vi "xy振镜移动-v2.vi"(0 "AO通道：X前Y后":tag="Dev1/ao0:1", 1 "f_scanlens(mm)":dbl=50.0, 2 "f_tubelens(mm)":dbl=200.0, 3 "f_objecitve(mm)":dbl=1.8, 5 "x终止位(um)":dbl=10.0, 7 "y终止位(um)":dbl=10.0, 9 "x初始位(um)":dbl, 11 "y初始位(um)":dbl, 12 "速度(um/s)":dbl=10.0, 13 "比例因子(V/°)":dbl=0.5) -> (6 "x终止位(um) 2":dbl=10.0, 8 "y终止位(um) 2":dbl=10.0)   [LabVIEW 2015]
doc: "速度为0时执行G0指令，可无需连接XY初始角"
uses:
  <vilib>/Platform/TimedLoop/XDataNode/timing_clust.ctl
  <vilib>/Platform/TimedLoop/XDataNode/nitl_modes.ctl
  <vilib>/Platform/TimedLoop/XDataNode/wakeup.ctl
  <vilib>/DAQmx/write.llb/DAQmx Write (Analog 1D DBL NChan 1Samp).vi
  <vilib>/DAQmx/write.llb/DAQmx Write (Analog DBL 1Chan 1Samp).vi
  <vilib>/DAQmx/create/channels.llb/DAQmx Create Channel (AO-Voltage-Basic).vi
  <vilib>/DAQmx/miscellaneous.llb/DAQmx Fill In Error Info.vi
  <vilib>/Platform/TimedLoop/XDataNode/XDataNode.xnode
  <vilib>/Platform/TimedLoop/XDataNode/XDNodeRunTimeDep.lvlib
panel:
  out "x当前角度(°)":dbl
  out "xy当前角度(°)":dbl[](array[numeric])
  out "y变压轨迹(°)":dbl[](array[numeric])=[0.0, 0.0, 0.002017457026776073, 0.006052371120349187, 0.012104742510839941, 0.020174571918626052, 0.030261861004579515, 0.042366612970385624, 0.05648883330894886, 0.07262853070489507, 0.09078571808518568, 0.11096041381986907, 0.13315264307300606, 0.15736243930382154, 0.1835898459181542, 0.21183491807029903, 0.24209772461536572, 0.27437835021230905, 0.30867689757782557, 0.3449934898913579, 0.38332827335149355, 0.42368141988411046, 0.46605313000267945, 0.5104436358212108, 0.5568532042204127, 0.6052821401677164, 0.6557307901919239, 0.7081995460133446, 0.7626888483303975, 0.819199190763796, 0.8777311239595615, 0.9382852598522744, 1.0008622760901253, 1.0654629206235144, 1.1320880164591356, 1.2007384665816805, 1.271415259045531, 1.3441194722390282, 1.4188522803241743, 1.495614958854875, 1.5744088905771372, 1.6552355714149243, 1.7380966166457146, 1.8229937672701457, 1.909928896580496, 1.998904016933165, 2.0899212867307106, 2.18298301761946, 2.2780916819091943, 2.375249920221874, 2.4744605493769543, 2.575726570521373, 2.6790511775129087, 2.784437765566249, 2.891889940171799, 3.0014115262979684, 3.1130065778884597, 3.226679387666904, 3.3424344972620594, 3.4602767076677168, 3.5802110900524586, 3.702242996935469, 3.826378073745729, 3.952622270783123, 4.080981855601287, 4.211463425833395, 4.344073922483553, 4.478820643708048, 4.615711259112385, 4.754753824591847, 4.895956797745277, 5.039329053893832, 5.18487990273871, 5.3326191056942776, 5.4825568939355716, 5.6347039872019975, 5.789071613401982, 5.94567152906667, 6.1045160407041665, 6.265618027109712, 6.428990962691198, 6.5946489418739285, 6.762606704653315, 6.932879663369455, 7.105483930783171, 7.2804363495393325, 7.4577545231099505, 7.6374568483168614, 7.819562549541885, 8.004091714740943, 8.19106533338831, 8.380505336487511, 8.572434638796867, 8.766877183430273, 8.963857989007577, 9.163403199544092, 9.365540137285489, 9.570297358712834, 9.777704713962741, 9.987793409930267, 10.200596077346972, 10.416146842154335, 10.634481401523217, 10.855637104904389, 11.079653040532992, 11.306570127852297, 11.536431216369454, 11.769281191509043, 12.00516708808958, 12.244138212115095, 12.486246271648975, 12.731545517622042, 12.980092895522644, 13.231948209024937, 13.487174296734457, 13.745837223369977, 14.008006486859884, 14.27375524301323, 14.543160549633939, 14.816303632185644, 15.09327017338965, 15.374150629455835, 15.659040576013455, 15.948041087234744, 16.241259152139953, 16.53880813265128, 16.84080826864106, 17.14738723601639, 17.45868076482219, 17.774833325457493, 18.095998892422205, 18.42234179659009, 18.754037678895433, 19.09127456059879, 19.434254048052267, 19.783192693234888, 20.13832353542236, 20.499897854386717, 20.868187171740544, 21.24348554477633, 21.62611220683683, 22.01641462046435, 22.4147720250887]
  out "x变压轨迹(°)":dbl[](array[numeric])=[0.0, 0.0, 0.002017457026776073, 0.006052371120349187, 0.012104742510839941, 0.020174571918626052, 0.030261861004579515, 0.042366612970385624, 0.05648883330894886, 0.07262853070489507, 0.09078571808518568, 0.11096041381986907, 0.13315264307300606, 0.15736243930382154, 0.1835898459181542, 0.21183491807029903, 0.24209772461536572, 0.27437835021230905, 0.30867689757782557, 0.3449934898913579, 0.38332827335149355, 0.42368141988411046, 0.46605313000267945, 0.5104436358212108, 0.5568532042204127, 0.6052821401677164, 0.6557307901919239, 0.7081995460133446, 0.7626888483303975, 0.819199190763796, 0.8777311239595615, 0.9382852598522744, 1.0008622760901253, 1.0654629206235144, 1.1320880164591356, 1.2007384665816805, 1.271415259045531, 1.3441194722390282, 1.4188522803241743, 1.495614958854875, 1.5744088905771372, 1.6552355714149243, 1.7380966166457146, 1.8229937672701457, 1.909928896580496, 1.998904016933165, 2.0899212867307106, 2.18298301761946, 2.2780916819091943, 2.375249920221874, 2.4744605493769543, 2.575726570521373, 2.6790511775129087, 2.784437765566249, 2.891889940171799, 3.0014115262979684, 3.1130065778884597, 3.226679387666904, 3.3424344972620594, 3.4602767076677168, 3.5802110900524586, 3.702242996935469, 3.826378073745729, 3.952622270783123, 4.080981855601287, 4.211463425833395, 4.344073922483553, 4.478820643708048, 4.615711259112385, 4.754753824591847, 4.895956797745277, 5.039329053893832, 5.18487990273871, 5.3326191056942776, 5.4825568939355716, 5.6347039872019975, 5.789071613401982, 5.94567152906667, 6.1045160407041665, 6.265618027109712, 6.428990962691198, 6.5946489418739285, 6.762606704653315, 6.932879663369455, 7.105483930783171, 7.2804363495393325, 7.4577545231099505, 7.6374568483168614, 7.819562549541885, 8.004091714740943, 8.19106533338831, 8.380505336487511, 8.572434638796867, 8.766877183430273, 8.963857989007577, 9.163403199544092, 9.365540137285489, 9.570297358712834, 9.777704713962741, 9.987793409930267, 10.200596077346972, 10.416146842154335, 10.634481401523217, 10.855637104904389, 11.079653040532992, 11.306570127852297, 11.536431216369454, 11.769281191509043, 12.00516708808958, 12.244138212115095, 12.486246271648975, 12.731545517622042, 12.980092895522644, 13.231948209024937, 13.487174296734457, 13.745837223369977, 14.008006486859884, 14.27375524301323, 14.543160549633939, 14.816303632185644, 15.09327017338965, 15.374150629455835, 15.659040576013455, 15.948041087234744, 16.241259152139953, 16.53880813265128, 16.84080826864106, 17.14738723601639, 17.45868076482219, 17.774833325457493, 18.095998892422205, 18.42234179659009, 18.754037678895433, 19.09127456059879, 19.434254048052267, 19.783192693234888, 20.13832353542236, 20.499897854386717, 20.868187171740544, 21.24348554477633, 21.62611220683683, 22.01641462046435, 22.4147720250887]
  out "移动次数":i32=142
  in  "AO通道：单通道":tag="Dev1/ao0:1"
  in  "dt(ms)":i32=10
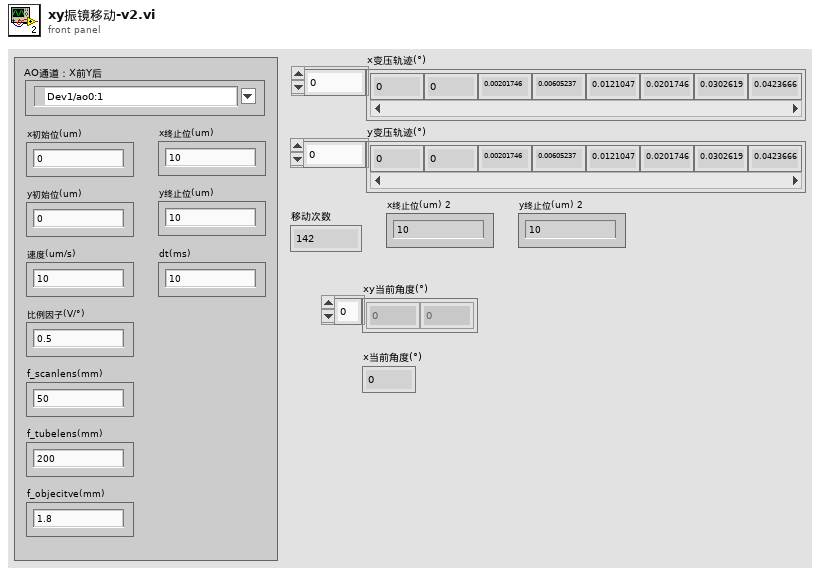
[diagram p1: front panel]
types:
  T1 = typedef "XDNodeRunTimeDep.lvlib/timing_clust.ctl" = cluster{"Expected End [f-1]":u64, "Actual End [f-1]":u64, "Finished Late? [f-1]":bool, "Expected End [i-1]":u64, "Actual End [i-1]":u64, "Finished Late? [i-1]":bool, "Expected Start [i]":u64, "Actual Start [i]":u64, "Expected Start [f]":u64, "Actual Start [f]":u64, "Source Name":string, "Structure Name":string, "Period":i64, "Deadline":i64, "Offset":i64, "Start":i64, "Priority":i32, "Timeout":i32, "Mode":T2, "Wakeup Reason":T3, "Error":errorcluster, "Source Type":string, "Secondary Source Type":string, "Global End Time":u64, "Global Start Time":u64, "Frame Duration":u64, "Iteration Duration":u64, "Assigned CPU":i32, "I/O Scan Engine Mode":u32}
  T2 = typedef "XDNodeRunTimeDep.lvlib/nitl_modes.ctl" = enum32{"No Change", "Process missed periods, maintain original phase", "Discard missed periods, maintain original phase", "Process missed periods, ignore original phase", "Discard missed periods, ignore original phase"}
  T3 = typedef "XDNodeRunTimeDep.lvlib/wakeup.ctl" = enum32{"Normal", "Aborted", "Asynchronous wakeup", "Timing source error", "Timed loop error", "Timeout"}
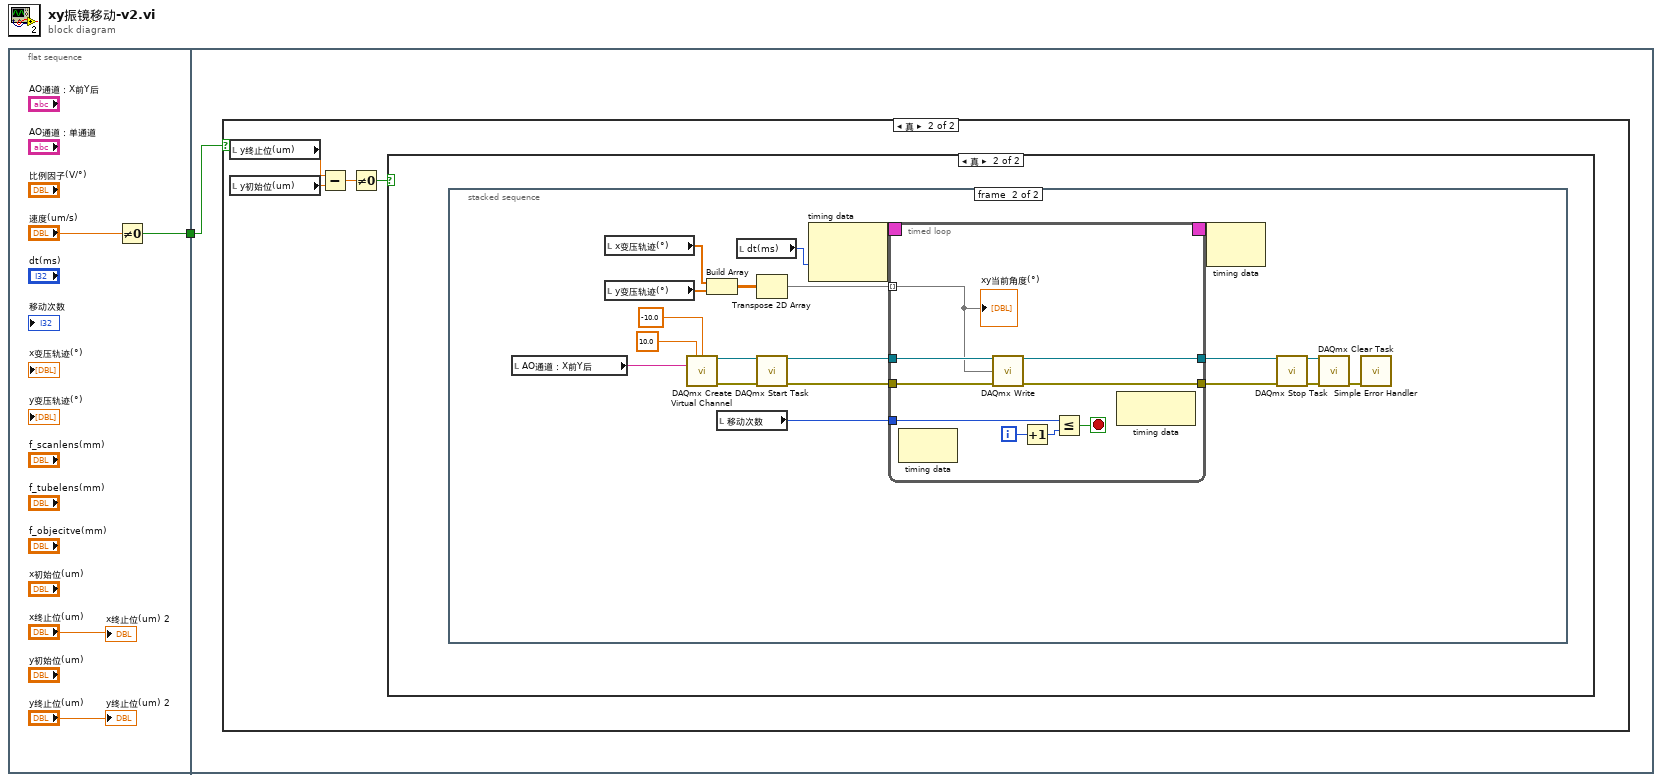
[diagram p0: block diagram]
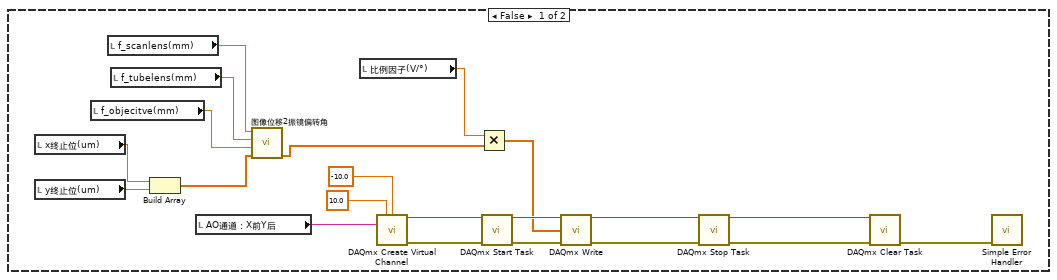
[diagram p2: hidden frame]
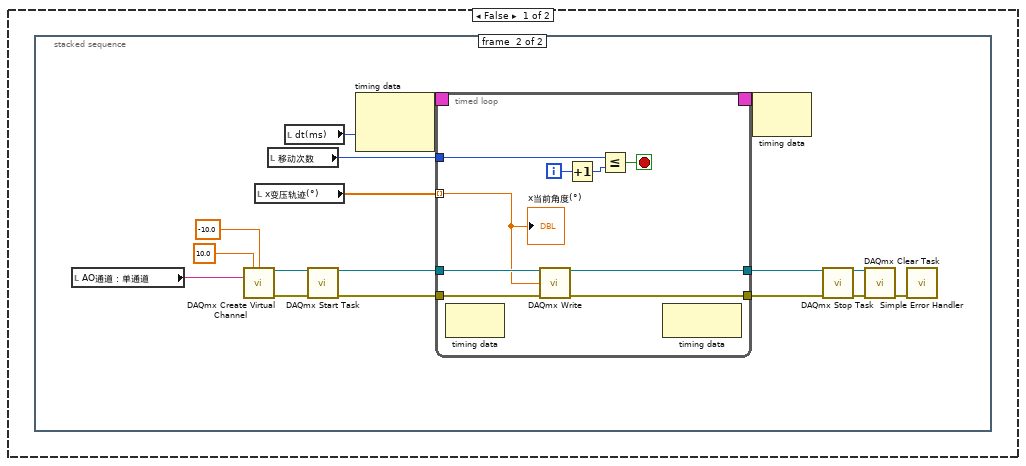
[diagram p3: hidden frame]
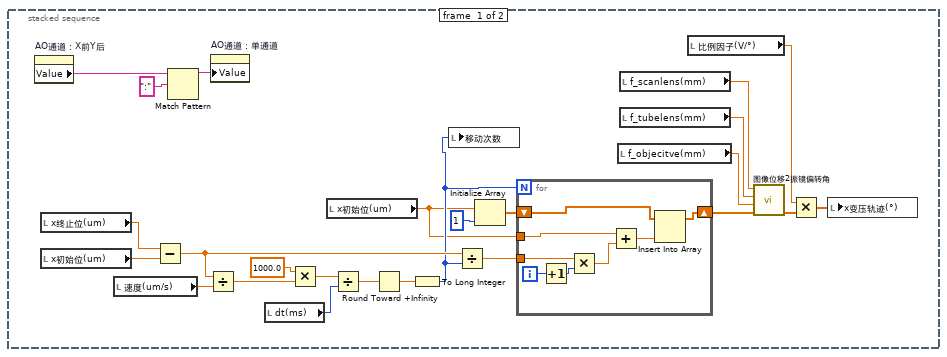
[diagram p4: hidden frame]
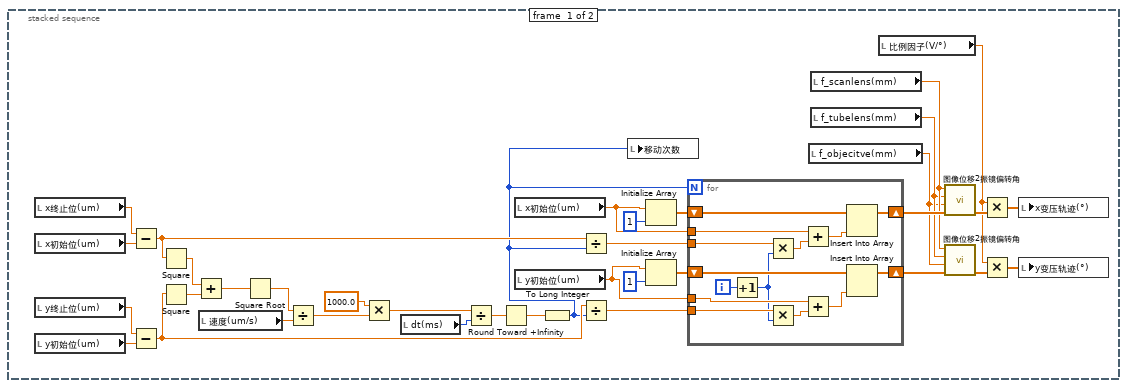
[diagram p5: hidden frame]
diagram:
  n1 = flat-sequence {
    tunnel: [w5] -> w1
    tunnel: w1 -> [w6]
    frame #0 {
      n2 = Not Equal To 0?(x="速度(um/s)") -> (x != 0?=w5:bool)
      "x终止位(um) 2" <- "x终止位(um)"
      "y终止位(um) 2" <- "y终止位(um)"
    }
    frame #1 {
      n3 = case shown="真" w6 {
        frame False {
          n4 = local read "x终止位(um)"() -> (w14:dbl)
          n5 = local read "y终止位(um)"() -> (w15:dbl)
          n6 = local read "f_objecitve(mm)"() -> (w9:dbl)
          n7 = local read "f_scanlens(mm)"() -> (w11:dbl)
          n8 = local read "f_tubelens(mm)"() -> (w10:dbl)
          n9 = Build Array(w14, w15) -> (w8:dbl[])
          n10 = local read "AO通道：X前Y后"() -> (w12:tag)
          n11 = call "图像位移2振镜偏转角.vi"("图像位移(um)"=w8, "f_objecitve(mm)"=w9, "f_tubelens(mm)"=w10, "f_scanlens(mm)"=w11) -> ("振镜偏转角(°)"=w7:dbl[])  [unwired: 7 in]
          n12 = local read "比例因子(V/°)"() -> (w13:dbl)
          n13 = call-poly <vilib>:"DAQmx Create Virtual Channel.vi"("maximum value"=10.0, "minimum value"=-10.0, "physical channels"=w12) -> ("task out"=w26:refnum<k21>, "error out"=w25:errorcluster)  [unwired: 11 in]
          n14 = Multiply(x=w13, y=w7) -> (x*y=w19:dbl[])
          n15 = call <vilib>:"DAQmx Start Task.vi"("task/channels in"=w26, "error in"=w25) -> ("task out"=w20:refnum<k21>, "error out"=w16:errorcluster)  [unwired: 12 in]
          n16 = call-poly <vilib>:"DAQmx Write.vi"("task/channels in"=w20, "data"=w19, "error in"=w16) -> ("task out"=w18:refnum<k21>, "error out"=w17:errorcluster)  [unwired: 10 in, 1 out]
          n17 = call <vilib>:"DAQmx Stop Task.vi"("task/channels in"=w18, "error in"=w17) -> ("task out"=w24:refnum<k21>, "error out"=w23:errorcluster)  [unwired: 12 in]
          n18 = call <vilib>:"DAQmx Clear Task.vi"("task in"=w24, "error in"=w23) -> ("error out"=w27:errorcluster)  [unwired: 13 in]
          n19 = call <vilib>:"Simple Error Handler.vi"("error in (no error)"=w27) -> ()  [unwired: 4 in, 5 out]
        }
        frame True {
          n20 = local read "y终止位(um)"() -> (w29:dbl)
          n21 = local read "y初始位(um)"() -> (w28:dbl)
          n22 = Subtract(x=w29, y=w28) -> (x-y=w31:dbl)
          n23 = Not Equal To 0?(x=w31) -> (x != 0?=w30:bool)
          n24 = case shown="真" w30 {
            frame False {
              n25 = stacked-sequence {
                frame #0 {
                  n26 = property on="AO通道：X前Y后" class="DAQmxName"() -> ("Value"=w54:string)  [unwired: 2 in, 2 out]
                  n27 = local read "x终止位(um)"() -> (w39:dbl)
                  n28 = local read "x初始位(um)"() -> (w41:dbl)
                  n29 = local read "速度(um/s)"() -> (w40:dbl)
                  n30 = Subtract(x=w39, y=w41) -> (x-y=w53:dbl)
                  n31 = Match Pattern(string=w54, regular expression=":" ("正则表达式")) -> (before substring=w56:string)  [unwired: 1 in, 3 out]
                  n32 = Divide(x=w53, y=w40) -> (x/y=w36:dbl)
                  n33 = property on="AO通道：单通道" class="DAQmxName"("Value"=w56) -> ()  [unwired: 2 in, 2 out]
                  n34 = local read "dt(ms)"() -> (w42:i32)
                  n35 = Multiply(x=1000.0, y=w36) -> (x*y=w38:dbl)
                  n36 = local read "x初始位(um)"() -> (w32:dbl)
                  n37 = Divide(x=w38, y=w42) -> (x/y=w34:dbl)
                  n38 = Round Toward +Infinity(x=w34) -> (ceil(x): smallest int >= x=w35:dbl)
                  n39 = To Long Integer(number=w35) -> (32bit integer=w33:i32)
                  n40 = local write "移动次数"(w33) -> ()
                  n41 = Divide(x=w53, y=w33) -> (x/y=w44:dbl)
                  n42 = Initialize Array(w32, 1 ("维数大小")) -> (w43:dbl[])
                  n43 = for {
                    N: w33 -> [_]
                    shift-right: [w60] -> w46
                    shift-left: w43 -> [w64]
                    tunnel: w44 -> [w63]
                    tunnel: w32 -> [w57]
                    i -> [w59]
                    n44 = Increment(x=w59) -> (x+1=w58:i32)
                    n45 = Multiply(x=w63, y=w58) -> (x*y=w62:dbl)
                    n46 = Add(x=w57, y=w62) -> (x+y=w61:dbl)
                    n47 = Insert Into Array(array=w64, new element=w61) -> (w60:dbl[])  [unwired: 1 in]
                  }
                  n48 = local read "f_objecitve(mm)"() -> (w49:dbl)
                  n49 = local read "f_scanlens(mm)"() -> (w47:dbl)
                  n50 = local read "f_tubelens(mm)"() -> (w48:dbl)
                  n51 = local read "比例因子(V/°)"() -> (w52:dbl)
                  n52 = call "图像位移2振镜偏转角.vi"("图像位移(um)"=w46, "f_objecitve(mm)"=w49, "f_tubelens(mm)"=w48, "f_scanlens(mm)"=w47) -> ("振镜偏转角(°)"=w50:dbl[])  [unwired: 7 in]
                  n53 = Multiply(x=w52, y=w50) -> (x*y=w51:dbl[])
                  n54 = local write "x变压轨迹(°)"(w51) -> ()
                }
                frame #1 {
                  n55 = local read "AO通道：单通道"() -> (w67:tag)
                  n56 = call-poly <vilib>:"DAQmx Create Virtual Channel.vi"("maximum value"=10.0, "minimum value"=-10.0, "physical channels"=w67) -> ("task out"=w78:refnum<k21>, "error out"=w77:errorcluster)  [unwired: 11 in]
                  n57 = local read "x变压轨迹(°)"() -> (w65:dbl[])
                  n58 = local read "移动次数"() -> (w66:i32)
                  n59 = local read "dt(ms)"() -> (w70:i32)
                  n60 = call <vilib>:"DAQmx Start Task.vi"("task/channels in"=w78, "error in"=w77) -> ("task out"=w76:refnum<k21>, "error out"=w75:errorcluster)  [unwired: 12 in]
                  n61 = node-c288(w70) -> (w81:T1)  [unwired: 1 in]
                  n62 = timed-loop {
                    tunnel: w76 -> [w90]
                    tunnel: w75 -> [w88]
                    tunnel: [w87] -> w73
                    tunnel: [w89] -> w74
                    timing: w81 -> [_]
                    timing-out: [_] -> w80
                    tunnel: w66 -> [w84]
                    tunnel: w65 -> [w82] mode=indexing
                    i -> [w86]
                    stop <- w83 stop-if-true
                    n63 = node-c288() -> ()  [unwired: 1 in, 1 out]
                    n64 = call-poly <vilib>:"DAQmx Write.vi"("task/channels in"=w90, "data"=w82, "error in"=w88) -> ("task out"=w89:refnum<k21>, "error out"=w87:errorcluster)  [unwired: 10 in, 1 out]
                    n65 = Increment(x=w86) -> (x+1=w85:i32)
                    n66 = Less Or Equal?(x=w84, y=w85) -> (x <= y?=w83:bool)
                    n67 = node-c288() -> ()  [unwired: 1 in, 1 out]
                    "x当前角度(°)" <- w82
                  }
                  n68 = node-c288(w80) -> ()  [unwired: 1 out]
                  n69 = call <vilib>:"DAQmx Stop Task.vi"("task/channels in"=w74, "error in"=w73) -> ("task out"=w72:refnum<k21>, "error out"=w71:errorcluster)  [unwired: 12 in]
                  n70 = call <vilib>:"DAQmx Clear Task.vi"("task in"=w72, "error in"=w71) -> ("error out"=w79:errorcluster)  [unwired: 13 in]
                  n71 = call <vilib>:"Simple Error Handler.vi"("error in (no error)"=w79) -> ()  [unwired: 4 in, 5 out]
                }
              }
            }
            frame True {
              n72 = stacked-sequence {
                frame #0 {
                  n73 = local read "x终止位(um)"() -> (w120:dbl)
                  n74 = local read "x初始位(um)"() -> (w117:dbl)
                  n75 = local read "y终止位(um)"() -> (w119:dbl)
                  n76 = local read "y初始位(um)"() -> (w121:dbl)
                  n77 = Subtract(x=w120, y=w117) -> (x-y=w122:dbl)
                  n78 = Subtract(x=w119, y=w121) -> (x-y=w123:dbl)
                  n79 = Square(x=w122) -> (x^2=w129:dbl)
                  n80 = Square(x=w123) -> (x^2=w130:dbl)
                  n81 = Add(x=w129, y=w130) -> (x+y=w131:dbl)
                  n82 = local read "速度(um/s)"() -> (w118:dbl)
                  n83 = Square Root(x=w131) -> (sqrt(x)=w132:dbl)
                  n84 = Divide(x=w132, y=w118) -> (x/y=w126:dbl)
                  n85 = Multiply(x=1000.0, y=w126) -> (x*y=w124:dbl)
                  n86 = local read "dt(ms)"() -> (w116:i32)
                  n87 = Divide(x=w124, y=w116) -> (x/y=w128:dbl)
                  n88 = Round Toward +Infinity(x=w128) -> (ceil(x): smallest int >= x=w127:dbl)
                  n89 = local read "x初始位(um)"() -> (w100:dbl)
                  n90 = local read "y初始位(um)"() -> (w101:dbl)
                  n91 = To Long Integer(number=w127) -> (32bit integer=w97:i32)
                  n92 = Divide(x=w122, y=w97) -> (x/y=w114:dbl)
                  n93 = Divide(x=w123, y=w97) -> (x/y=w113:dbl)
                  n94 = local write "移动次数"(w97) -> ()
                  n95 = Initialize Array(w100, 1 ("维数大小")) -> (w115:dbl[])
                  n96 = Initialize Array(w101, 1 ("维数大小")) -> (w112:dbl[])
                  n97 = for {
                    N: w97 -> [_]
                    shift-right: [w137] -> w111
                    shift-left: w115 -> [w146]
                    tunnel: w114 -> [w144]
                    tunnel: w113 -> [w143]
                    shift-right: [w138] -> w110
                    shift-left: w112 -> [w145]
                    tunnel: w100 -> [w136]
                    tunnel: w101 -> [w135]
                    i -> [w134]
                    n98 = Increment(x=w134) -> (x+1=w133:i32)
                    n99 = Multiply(x=w144, y=w133) -> (x*y=w141:dbl)
                    n100 = Multiply(x=w143, y=w133) -> (x*y=w142:dbl)
                    n101 = Add(x=w136, y=w141) -> (x+y=w140:dbl)
                    n102 = Add(x=w135, y=w142) -> (x+y=w139:dbl)
                    n103 = Insert Into Array(array=w146, new element=w140) -> (w137:dbl[])  [unwired: 1 in]
                    n104 = Insert Into Array(array=w145, new element=w139) -> (w138:dbl[])  [unwired: 1 in]
                  }
                  n105 = local read "f_objecitve(mm)"() -> (w107:dbl)
                  n106 = local read "f_scanlens(mm)"() -> (w109:dbl)
                  n107 = local read "f_tubelens(mm)"() -> (w108:dbl)
                  n108 = local read "比例因子(V/°)"() -> (w103:dbl)
                  n109 = call "图像位移2振镜偏转角.vi"("图像位移(um)"=w111, "f_objecitve(mm)"=w107, "f_tubelens(mm)"=w108, "f_scanlens(mm)"=w109) -> ("振镜偏转角(°)"=w106:dbl[])  [unwired: 7 in]
                  n110 = call "图像位移2振镜偏转角.vi"("图像位移(um)"=w110, "f_objecitve(mm)"=w107, "f_tubelens(mm)"=w108, "f_scanlens(mm)"=w109) -> ("振镜偏转角(°)"=w104:dbl[])  [unwired: 7 in]
                  n111 = Multiply(x=w103, y=w106) -> (x*y=w105:dbl[])
                  n112 = Multiply(x=w103, y=w104) -> (x*y=w102:dbl[])
                  n113 = local write "x变压轨迹(°)"(w105) -> ()
                  n114 = local write "y变压轨迹(°)"(w102) -> ()
                }
                frame #1 {
                  n115 = local read "AO通道：X前Y后"() -> (w152:tag)
                  n116 = local read "x变压轨迹(°)"() -> (w150:dbl[])
                  n117 = local read "y变压轨迹(°)"() -> (w149:dbl[])
                  n118 = call-poly <vilib>:"DAQmx Create Virtual Channel.vi"("maximum value"=10.0, "minimum value"=-10.0, "physical channels"=w152) -> ("task out"=w163:refnum<k21>, "error out"=w162:errorcluster)  [unwired: 11 in]
                  n119 = Build Array(w150, w149) -> (w148:dbl[][])
                  n120 = local read "移动次数"() -> (w151:i32)
                  n121 = local read "dt(ms)"() -> (w155:i32)
                  n122 = Transpose 2D Array(2D array=w148) -> (transposed array=w147:dbl[][])
                  n123 = call <vilib>:"DAQmx Start Task.vi"("task/channels in"=w163, "error in"=w162) -> ("task out"=w161:refnum<k21>, "error out"=w160:errorcluster)  [unwired: 12 in]
                  n124 = node-c288(w155) -> (w166:T1)  [unwired: 1 in]
                  n125 = timed-loop {
                    tunnel: w161 -> [w175]
                    tunnel: w160 -> [w173]
                    tunnel: [w172] -> w158
                    tunnel: [w174] -> w159
                    timing: w166 -> [_]
                    timing-out: [_] -> w165
                    tunnel: w151 -> [w168]
                    tunnel: w147 -> [w167] mode=indexing
                    i -> [w171]
                    stop <- w169 stop-if-true
                    n126 = node-c288() -> ()  [unwired: 1 in, 1 out]
                    n127 = call-poly <vilib>:"DAQmx Write.vi"("task/channels in"=w175, "data"=w167, "error in"=w173) -> ("task out"=w174:refnum<k21>, "error out"=w172:errorcluster)  [unwired: 10 in, 1 out]
                    n128 = Increment(x=w171) -> (x+1=w170:i32)
                    n129 = Less Or Equal?(x=w168, y=w170) -> (x <= y?=w169:bool)
                    n130 = node-c288() -> ()  [unwired: 1 in, 1 out]
                    "xy当前角度(°)" <- w167
                  }
                  n131 = node-c288(w165) -> ()  [unwired: 1 out]
                  n132 = call <vilib>:"DAQmx Stop Task.vi"("task/channels in"=w159, "error in"=w158) -> ("task out"=w157:refnum<k21>, "error out"=w156:errorcluster)  [unwired: 12 in]
                  n133 = call <vilib>:"DAQmx Clear Task.vi"("task in"=w157, "error in"=w156) -> ("error out"=w164:errorcluster)  [unwired: 13 in]
                  n134 = call <vilib>:"Simple Error Handler.vi"("error in (no error)"=w164) -> ()  [unwired: 4 in, 5 out]
                }
              }
            }
          }
        }
      }
    }
  }
